vi "analyseData.vi"(8 "error in (no error)":errorcluster, 10 "HGF_VariantDataObject in":refnum<class "HGF_VariantDataObject.lvclass">, 11 "WfmAnalysator in":refnum<class "WfmAnalysator.lvclass">) -> (0 "error out":errorcluster, 2 "HGF_VariantDataObject out":refnum<class "HGF_VariantDataObject.lvclass">, 3 "WfmAnalysator out":refnum<class "WfmAnalysator.lvclass">)   [LabVIEW 2012, in "MyApp.lvlib" / "WfmAnalysator.lvclass"]
doc: "Analyse data contained in HGF_DataVariantObject by using the HGF_DataAnalysator objects and optionally compining their results for a summaray result.\n\nThis is a dynamic dispatch VI to be overwritten by child classes."
uses:
  WfmAnalysator.lvclass
  HGF_LVC/HGF_BaseClasses/HGF_VariantDataObject/HGF_VariantDataObject.lvclass
  Wfm_Amplitude/Wfm_Amplitude.lvclass
  Wfm_PulseMeasurement/Wfm_PulseMeasurement.lvclass
  HGF_DataAnalysator/HGF_DataAnalysator.lvclass
  WfmAnalysator.lvclass/WfmAnalysator.ctl
  HGF_LVC/HGF_BaseClasses/HGF_Composite/HGF_Composite.lvclass
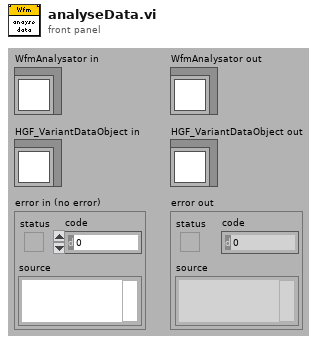
[diagram p1: front panel]
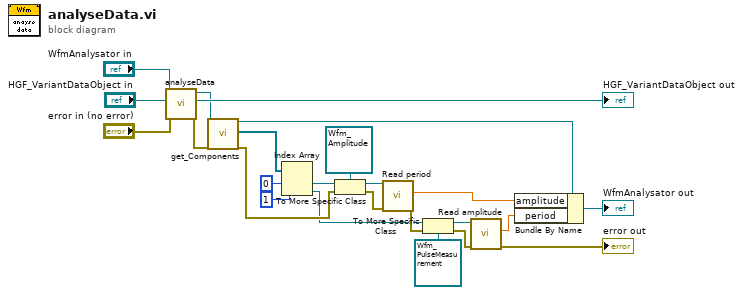
[diagram p0: block diagram]
diagram:
  n1 = call-parent "analyseData.vi"("error in (no error)"="error in (no error)", "HGF_VariantDataObject in"="HGF_VariantDataObject in", "HGF_DataAnalysator in"="WfmAnalysator in") -> ("error out"=w14:errorcluster, "HGF_VariantDataObject out"=→"HGF_VariantDataObject out":refnum<class "HGF_VariantDataObject.lvclass">, "HGF_DataAnalysator out"=w15:refnum<class "WfmAnalysator.lvclass">)  [unwired: 6 in]
  n2 = call "get_Components.vi"("HGF_Composite"=w15, "error in (no error)"=w14) -> ("dup HGF_Composite"=w12:refnum<class "WfmAnalysator.lvclass">, "Components"=w13:refnum<class "HGF_Component.lvclass">[], "error out"=w9:errorcluster)  [unwired: 15 in]
  n3 = Index Array(array=w13, index #1=0 ("index"), index #2=1 ("index")) -> (element #1=w2:refnum<class "HGF_Component.lvclass">, element #2=w1:refnum<class "HGF_Component.lvclass">)
  n4 = To More Specific Class(target class=refnum<class "Wfm_Amplitude.lvclass"> refnum ("MyApp.lvlib:Wfm_Amplitude.lvclass"), reference=w2, error in=w9) -> (specific class reference=w7:refnum<class "Wfm_Amplitude.lvclass">, error out=w6:errorcluster)
  n5 = call "Read period.vi"("error in (no error)"=w6, "Wfm_Amplitude in"=w7) -> ("error out"=w4:errorcluster, "amplitude"=w5:dbl)  [unwired: 5 in, 3 out]
  n6 = To More Specific Class(target class=refnum<class "Wfm_PulseMeasurement.lvclass"> refnum ("MyApp.lvlib:Wfm_PulseMeasurement.lvclass"), reference=w1, error in=w4) -> (specific class reference=w16:refnum<class "Wfm_PulseMeasurement.lvclass">, error out=w10:errorcluster)
  n7 = call "Read amplitude.vi"("error in (no error)"=w10, "Wfm_PulseMeasurement in"=w16) -> ("error out"=→"error out":errorcluster, "period"=w3:dbl)  [unwired: 4 in, 4 out]
  n8 = Bundle By Name(cluster=w12, "amplitude"=w5, "period"=w3) -> (→"WfmAnalysator out":refnum<class "WfmAnalysator.lvclass">)
